vi "FTW-JSON-Core-Serialize.vi"(0 "JSON Object":i64 format="%016x", 5 "Encoding Flags":i64 format="%016x", 11 "error in":errorcluster) -> (4 "JSON Object":i64 format="%016x", 6 "JSON String (UTF-8)":string, 15 "error out":errorcluster)   [LabVIEW 2015, in "FTW-JSON.lvclass"]
uses:
  FTW-JSON.lvclass
panel:
  # "Inputs"
  # "Outputs"
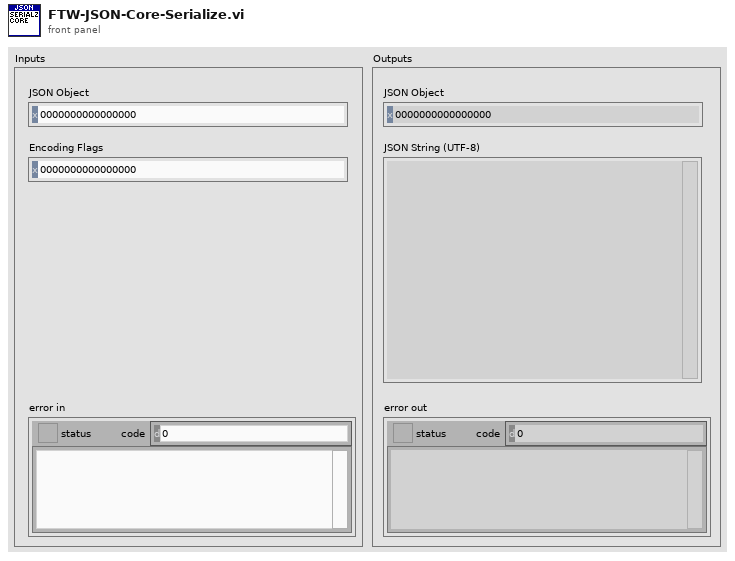
[diagram p1: front panel]
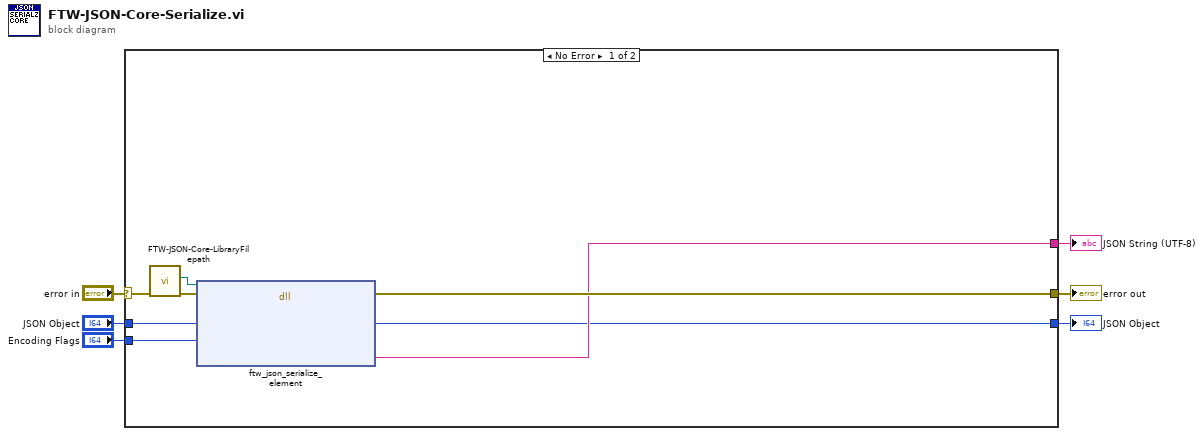
[diagram p0: block diagram]
diagram:
  n1 = case shown="No Error" "error in" {
    selector: "error in" -> [w14 w16]
    tunnel: [w11 w16] -> w6
    tunnel: [w7 w15] -> w4
    tunnel: "JSON Object" -> [w9 w15]
    tunnel: [w10 _] -> w2
    tunnel: "Encoding Flags" -> [w8 _]
    frame No Error {
      n2 = call "FTW-JSON-Core-LibraryFilepath.vi"("error in"=w14) -> ("error out"=w13:errorcluster, "JSON Library Filepath"=w12:path)  [unwired: 9 in]
      n3 = dll-call lib="?" fn="ftw_json_serialize_element"(path in=w12, error in=w13, "JSON Object Pointer"=w9, "Flags"=w8) -> (error out=w11:errorcluster, "JSON Object Pointer"=w7:i64, "Serialized String"=w10:string)  [unwired: 4 in, 1 out]
    }
    frame Error {
    }
  }
  "error out" <- w6
  "JSON Object" <- w4
  "JSON String (UTF-8)" <- w2
